vi "Get Slider Value.vi"(7 "Logarithm?":bool, 9 "Bottom Numeric":sgl, 10 "Top Numeric":sgl, 11 "Current Numeric":sgl) -> (3 "Current Slider":i32)   [LabVIEW 2020, in "3D Plot.lvclass"]
uses:
  3D Plot.lvclass
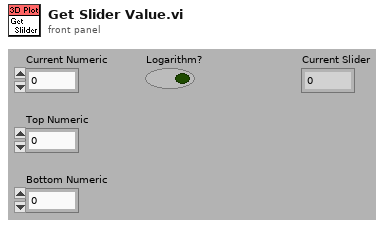
[diagram p1: front panel]
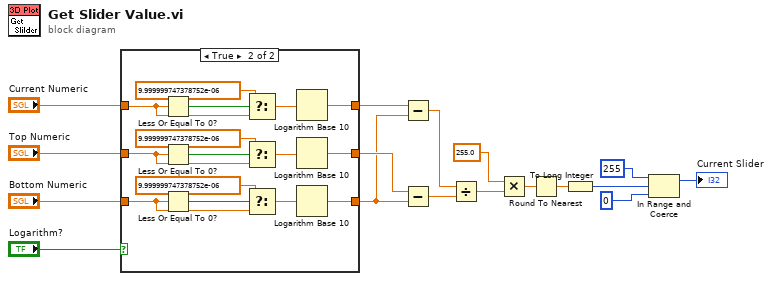
[diagram p0: block diagram]
diagram:
  n1 = case shown="True" "Logarithm?" {
    tunnel: [w20 w33] -> w7
    tunnel: "Current Numeric" -> [w20 w22]
    tunnel: [w19 w35] -> w9
    tunnel: "Top Numeric" -> [w19 w21]
    tunnel: [w18 w34] -> w5
    tunnel: "Bottom Numeric" -> [w18 w30]
    frame False {
    }
    frame True {
      n2 = Less Or Equal To 0?(x=w22) -> (x <= 0?=w28:bool)
      n3 = Less Or Equal To 0?(x=w21) -> (x <= 0?=w26:bool)
      n4 = Less Or Equal To 0?(x=w30) -> (x <= 0?=w32:bool)
      n5 = Select(t=sgl 1e-05, s=w28, f=w22) -> (s? t:f=w23:sgl)
      n6 = Select(t=sgl 1e-05, s=w26, f=w21) -> (s? t:f=w24:sgl)
      n7 = Select(t=sgl 1e-05, s=w32, f=w30) -> (s? t:f=w29:sgl)
      n8 = Logarithm Base 10(1:w23) -> (0:w33:sgl)
      n9 = Logarithm Base 10(1:w24) -> (0:w35:sgl)
      n10 = Logarithm Base 10(1:w29) -> (0:w34:sgl)
    }
  }
  n11 = Subtract(x=w7, y=w5) -> (x-y=w6:sgl)
  n12 = Subtract(x=w9, y=w5) -> (x-y=w13:sgl)
  n13 = Divide(x=w6, y=w13) -> (x/y=w8:sgl)
  n14 = Multiply(x=sgl 255.0 ("y"), y=w8) -> (x*y=w12:sgl)
  n15 = Round To Nearest(number=w12) -> (nearest integer value=w11:sgl)
  n16 = To Long Integer(number=w11) -> (32bit integer=w4:i32)
  n17 = In Range and Coerce(upper limit=255, x=w4, lower limit=0) -> (coerced(x)=→"Current Slider":i32)  [unwired: 1 out]
